vi "ZeroMQ_FOC_REQREP.vi"() -> ()   [LabVIEW 2018]
uses:
  <vilib>/addons/zeromq/socket_type.ctl
  <vilib>/addons/zeromq/socket_options.ctl
  <vilib>/addons/zeromq/zeromq.lvlib
  <vilib>/addons/zeromq/zmq_socket.lvclass
  <vilib>/addons/zeromq/zmq_context.lvclass
panel:
  out "error out 3":errorcluster
  out "error out 4":errorcluster
  in  "stop 4":bool
  out "command 2":string
  out "reply":string
  out "error out 2":errorcluster
  out "message":string
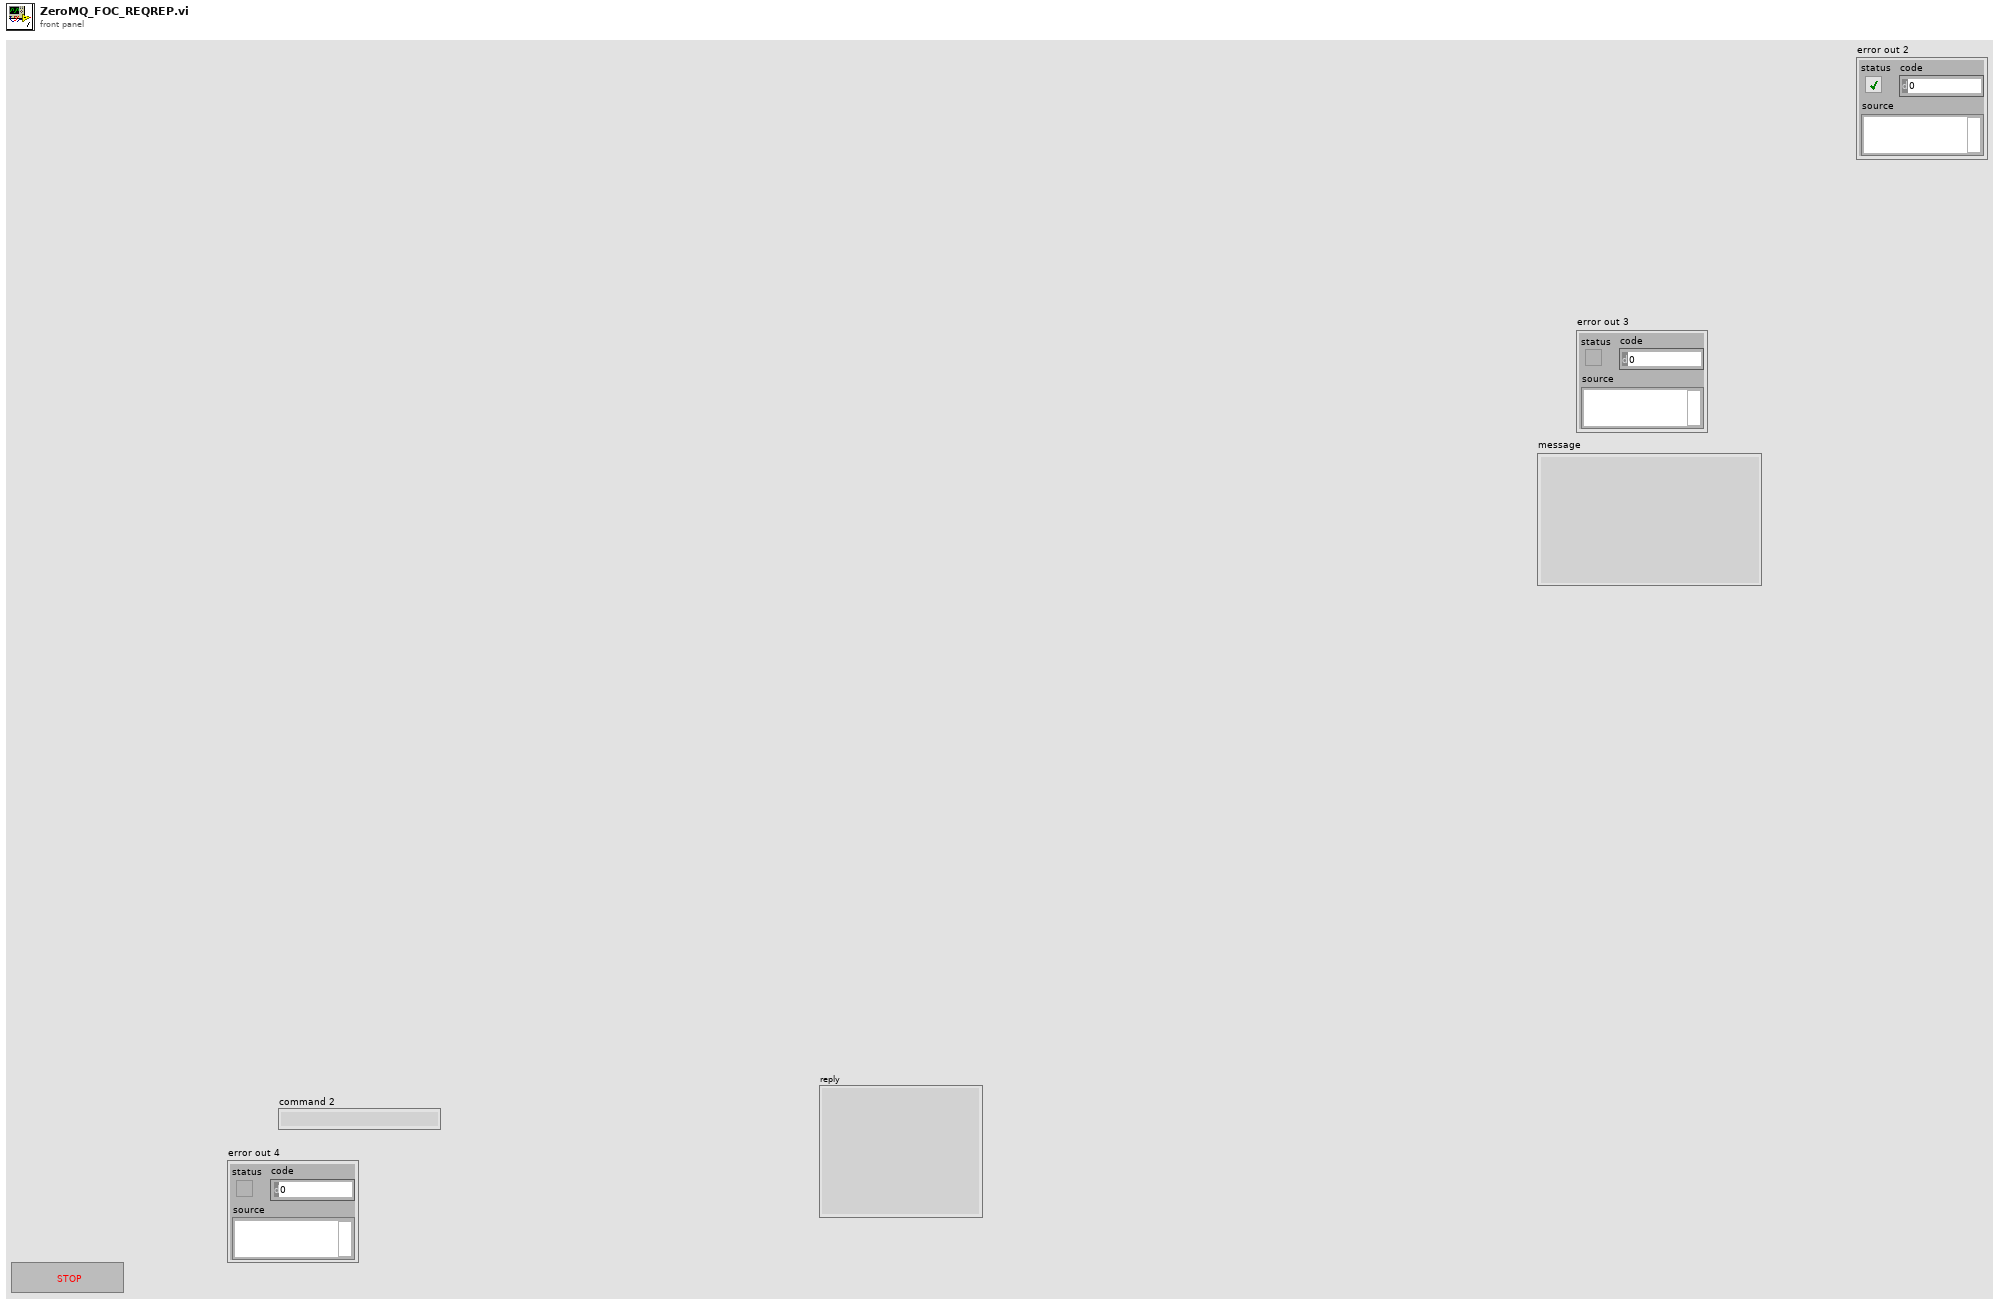
[diagram p1: front panel]
types:
  T1 = typedef "zeromq.lvlib/socket_options.ctl" = enum8{"NONE", "ZMQ_HWM", "<2>", "ZMQ_SWAP", "ZMQ_AFFINITY", "ZMQ_ROUTING_ID", "ZMQ_SUBSCRIBE", "ZMQ_UNSUBSCRIBE", "ZMQ_RATE", "ZMQ_RECOVERY_IVL", "ZMQ_MCAST_LOOP", "ZMQ_SNDBUF", "ZMQ_RCVBUF", "ZMQ_RCVMORE", "ZMQ_FD", "ZMQ_EVENTS", "ZMQ_TYPE", "ZMQ_LINGER", "ZMQ_RECONNECT_IVL", "ZMQ_BACKLOG", "ZMQ_RECOVERY_IVL_MSEC", "ZMQ_RECONNECT_IVL_MAX", "ZMQ_MAXMSGSIZE", "ZMQ_SNDHWM", "ZMQ_RCVHWM", "ZMQ_MULTICAST_HOPS", "<26>", "ZMQ_RCVTIMEO", "ZMQ_SNDTIMEO", "<29>", "<30>", "ZMQ_IPV4ONLY", "ZMQ_LAST_ENDPOINT", "ZMQ_ROUTER_MANDATORY", "ZMQ_TCP_KEEPALIVE", "ZMQ_TCP_KEEPALIVE_CNT", "ZMQ_TCP_KEEPALIVE_IDLE", "ZMQ_TCP_KEEPALIVE_INTVL", "ZMQ_TCP_ACCEPT_FILTER", "ZMQ_IMMEDIATE", "ZMQ_XPUB_VERBOSE", "ZMQ_ROUTER_RAW", "ZMQ_IPV6", "ZMQ_MECHANISM", "ZMQ_PLAIN_SERVER", "ZMQ_PLAIN_USERNAME", "ZMQ_PLAIN_PASSWORD", "ZMQ_CURVE_SERVER", "ZMQ_CURVE_PUBLICKEY", "ZMQ_CURVE_SECRETKEY", "ZMQ_CURVE_SERVERKEY", "ZMQ_PROBE_ROUTER", "ZMQ_REQ_CORRELATE", "ZMQ_REQ_RELAXED", "ZMQ_CONFLATE", "ZMQ_ZAP_DOMAIN", "ZMQ_ROUTER_HANDOVER", "ZMQ_TOS", "ZMQ_IPC_FILTER_PID", "ZMQ_IPC_FILTER_UID", "ZMQ_IPC_FILTER_GID", "ZMQ_CONNECT_ROUTING_ID", "ZMQ_GSSAPI_SERVER", "ZMQ_GSSAPI_PRINCIPAL", "ZMQ_GSSAPI_SERVICE_PRINCIPAL", "ZMQ_GSSAPI_PLAINTEXT", "ZMQ_HANDSHAKE_IVL", "<67>", "ZMQ_SOCKS_PROXY", "ZMQ_XPUB_NODROP", "ZMQ_BLOCKY", "ZMQ_XPUB_MANUAL", "ZMQ_XPUB_WELCOME_MSG", "ZMQ_STREAM_NOTIFY", "ZMQ_INVERT_MATCHING", "ZMQ_HEARTBEAT_IVL", "ZMQ_HEARTBEAT_TTL", "ZMQ_HEARTBEAT_TIMEOUT", "ZMQ_XPUB_VERBOSER", "ZMQ_CONNECT_TIMEOUT", "ZMQ_TCP_MAXRT", "ZMQ_THREAD_SAFE", "<82>", "<83>", "ZMQ_MULTICAST_MAXTPDU", "ZMQ_VMCI_BUFFER_SIZE", "ZMQ_VMCI_BUFFER_MIN_SIZE", "ZMQ_VMCI_BUFFER_MAX_SIZE", "ZMQ_VMCI_CONNECT_TIMEOUT", "ZMQ_USE_FD", "ZMQ_GSSAPI_PRINCIPAL_NAMETYPE", "ZMQ_GSSAPI_SERVICE_PRINCIPAL_NAMETYPE", "ZMQ_BINDTODEVICE", "ZMQ_ZAP_ENFORCE_DOMAIN", "ZMQ_LOOPBACK_FASTPATH", "ZMQ_METADATA", "ZMQ_MULTICAST_LOOP", "ZMQ_ROUTER_NOTIFY"}
  T2 = typedef "zeromq.lvlib/socket_type.ctl" = enum8{"ZMQ_PAIR", "ZMQ_PUB", "ZMQ_SUB", "ZMQ_REQ", "ZMQ_REP", "ZMQ_DEALER", "ZMQ_ROUTER", "ZMQ_PULL", "ZMQ_PUSH", "ZMQ_XPUB", "ZMQ_XSUB", "ZMQ_STREAM", "ZMQ_SERVER", "ZMQ_CLIENT", "ZMQ_RADIO", "ZMQ_DISH", "ZMQ_GATHER", "ZMQ_SCATTER", "ZMQ_DGRAM"}
  T3 = cluster{"ID":u32, "Address":string, "Service Name 1":string, "Service Name 2":string, "queue TX":refnum<queue>, "queue RX":refnum<queue>, "Port 1":u32, "Port 2":u32}
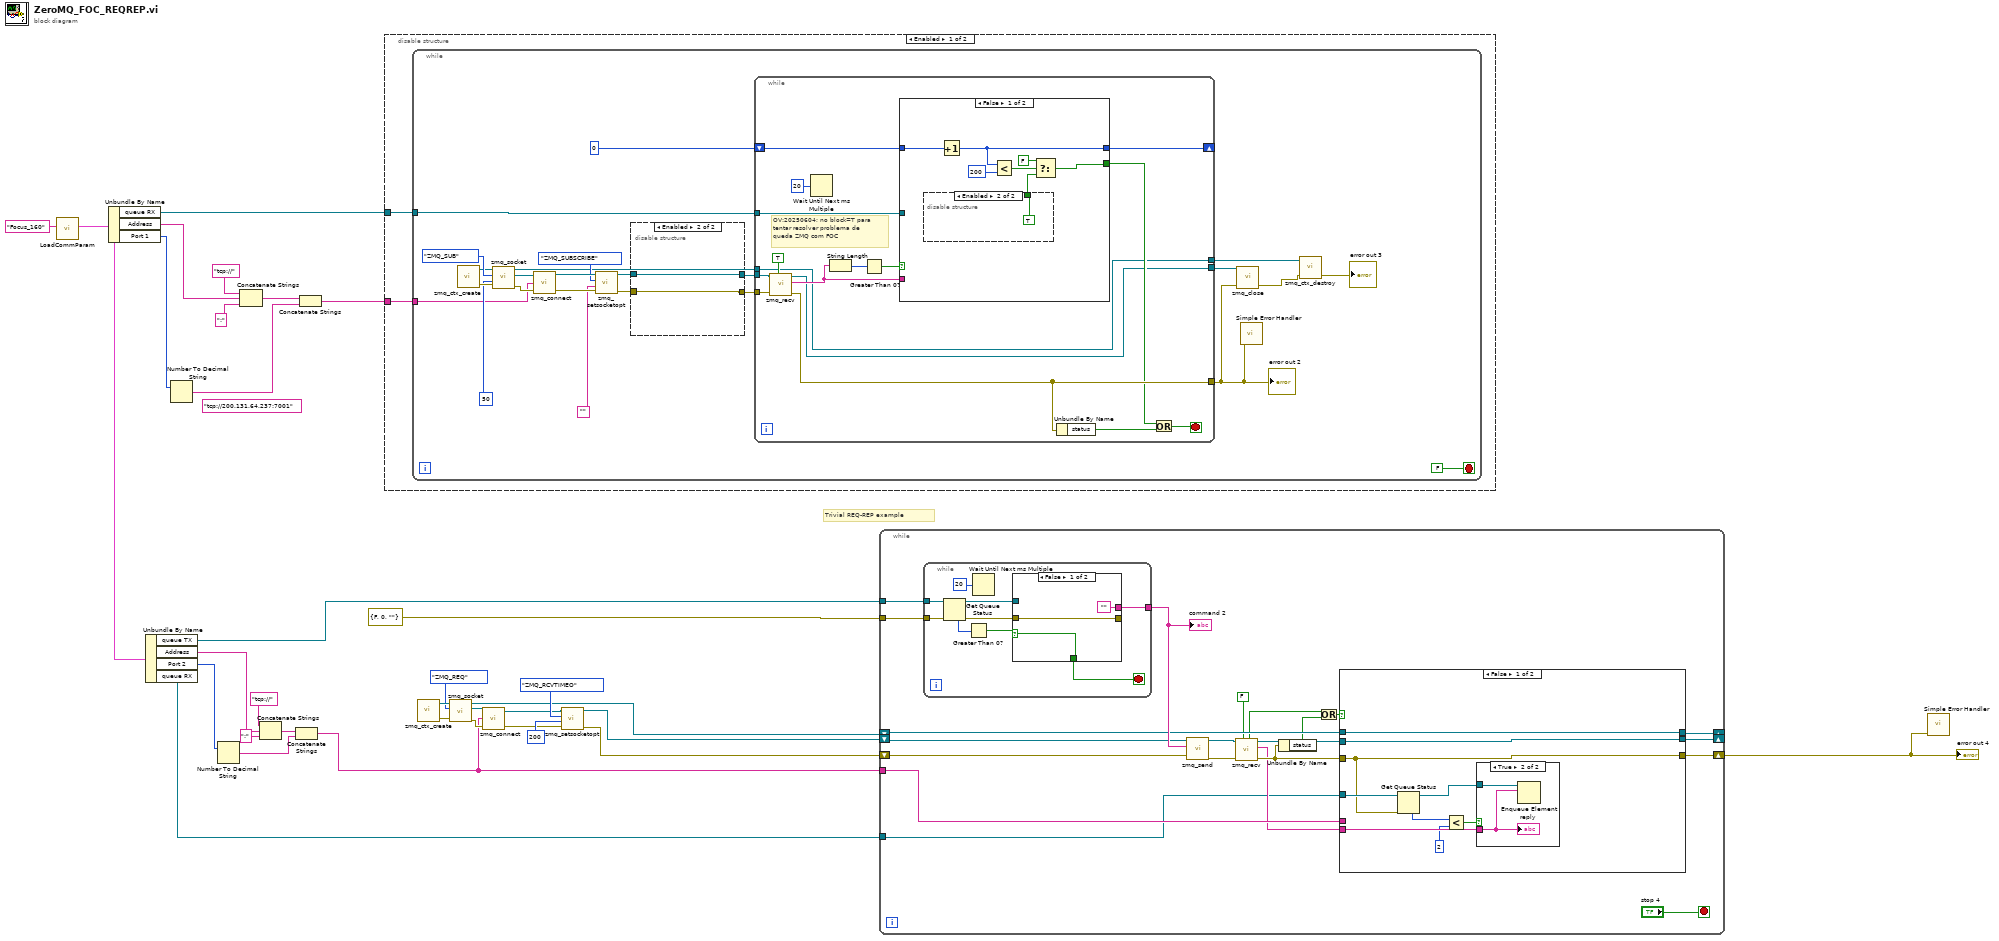
[diagram p0: block diagram]
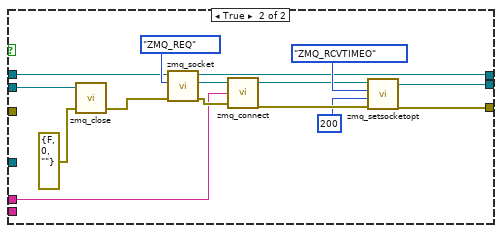
[diagram p3: hidden frame]
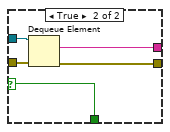
[diagram p4: hidden frame]
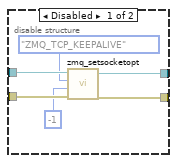
[diagram p5: hidden frame]
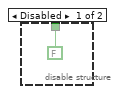
[diagram p6: hidden frame]
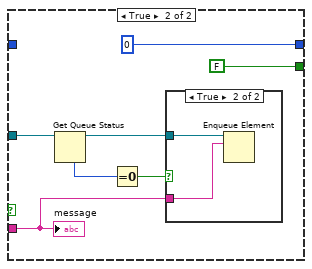
[diagram p7: hidden frame]
diagram:
  (unwired) "tcp://200.131.64.237:7001" ("endpoint")
  # "Trivial REQ-REP example"
  n1 = call "LoadCommParam.vi"("section name"="Focus_160") -> ("output cluster"=w1:T3)  [unwired: 10 in]
  n2 = Unbundle By Name(w1) -> ("queue RX"=w25:refnum<queue>, "Address"=w32:string, "Port 1"=w31:u32)
  n3 = Unbundle By Name(w1) -> ("queue TX"=w16:refnum<queue>, "Address"=w18:string, "Port 2"=w17:u32, "queue RX"=w2:refnum<queue>)
  n4 = Number To Decimal String(number=w31) -> (decimal integer string=w30:string)  [unwired: 1 in]
  n5 = Number To Decimal String(number=w17) -> (decimal integer string=w22:string)  [unwired: 1 in]
  n6 = Concatenate Strings("tcp://" ("string"), w32, ":" ("string")) -> (w29:string)
  n7 = Concatenate Strings("tcp://" ("string"), w18, ":" ("string")) -> (w21:string)
  n8 = Concatenate Strings(w21, w22) -> (w10:string)
  n9 = Concatenate Strings(w29, w30) -> (w26:string)
  n10 = disable-structure shown="Enabled" {
    disable-tunnel: w25 -> [w35 _]
    disable-tunnel: w26 -> [w34 _]
    frame Enabled {
      n11 = while {
        tunnel: w35 -> [w50]
        tunnel: w34 -> [w49]
        stop <- FALSE stop-if-true
        n12 = call <vilib>:"zmq_ctx_create.vi"() -> ("error out"=w58:errorcluster, "context out"=w52:refnum<class "zmq_context.lvclass">)  [unwired: 4 in]
        n13 = call <vilib>:"zmq_socket.vi"("error in"=w58, "linger (ms)"=50, "socket type"=socket_type."ZMQ_SUB", "context in"=w52) -> ("error out"=w57:errorcluster, "socket out"=w53:refnum<class "zmq_socket.lvclass">, "context out"=w41:refnum<class "zmq_context.lvclass">)  [unwired: 1 in]
        n14 = call <vilib>:"zmq_connect.vi"("error in"=w57, "endpoint"=w49, "socket in"=w53) -> ("error out"=w55:errorcluster, "socket out"=w56:refnum<class "zmq_socket.lvclass">)  [unwired: 1 in]
        n15 = call <vilib>:"zmq_setsocketopt.vi"("error in"=w55, "value"="", "option"=socket_options."ZMQ_SUBSCRIBE", "socket in"=w56) -> ("error out"=w44:errorcluster, "socket out"=w46:refnum<class "zmq_socket.lvclass">)  [unwired: 2 in]
        n16 = disable-structure shown="Enabled" {
          disable-tunnel: w46 -> [w65 w67]
          disable-tunnel: [w64 w67] -> w45
          disable-tunnel: w44 -> [w63 w66]
          disable-tunnel: [w62 w66] -> w43
          frame Disabled {
            n17 = call <vilib>:"zmq_setsocketopt.vi"("error in"=w63, "value"=-1, "option"=socket_options."ZMQ_TCP_KEEPALIVE", "socket in"=w65) -> ("error out"=w62:errorcluster, "socket out"=w64:refnum<class "zmq_socket.lvclass">)  [unwired: 2 in]
          }
          frame Enabled {
          }
        }
        n18 = while {
          tunnel: w45 -> [w82]
          tunnel: w43 -> [w83]
          tunnel: [w73] -> w38
          tunnel: w50 -> [w79]
          shift-right: [w74] -> _
          shift-left: 0 -> [w75]
          tunnel: [w69] -> w40
          tunnel: w41 -> [w68]
          tunnel: [w68] -> w39
          stop <- w70 stop-if-true
          # "OV:20250604; no block=T para\ntentar resolver problema de\nqueda ZMQ com FOC"
          n19 = call <vilib>:"zmq_recv.vi"("no block? (F)"=TRUE, "error in"=w83, "socket in"=w82) -> ("error out"=w73:errorcluster, "data"=w78:string, "socket out"=w69:refnum<class "zmq_socket.lvclass">)  [unwired: 2 in, 2 out]
          n20 = Wait Until Next ms Multiple(millisecond multiple=u32 20) -> ()  [unwired: 1 out]
          n21 = String Length(string=w78) -> (length=w81:i32)
          n22 = Greater Than 0?(x=w81) -> (x > 0?=w80:bool)
          n23 = case shown="False" w80 {
            tunnel: w79 -> [_ w98]
            tunnel: w78 -> [_ w95]
            tunnel: w75 -> [w90 _]
            tunnel: [w89 0] -> w74
            tunnel: [w86 FALSE] -> w71
            frame False {
              n24 = disable-structure shown="Enabled" {
                disable-tunnel: [FALSE ("f") TRUE] -> w84
                frame Disabled {
                }
                frame Enabled {
                }
              }
              n25 = Increment(x=w90) -> (x+1=w89:i32)
              n26 = Less?(x=w89, y=200) -> (x < y?=w87:bool)
              n27 = Select(t=FALSE, s=w87, f=w84) -> (s? t:f=w86:bool)
            }
            frame True {
              n28 = Get Queue Status(queue=w98) -> (queue out=w96:refnum<queue>, # elements in queue=w99:i32)  [unwired: 2 in, 6 out]
              n29 = Equal To 0?(x=w99) -> (x = 0?=w97:bool)
              n30 = case shown="True" w97 {
                tunnel: w96 -> [_ w101]
                tunnel: w95 -> [_ w100]
                frame False {
                }
                frame True {
                  n31 = Enqueue Element(queue=w101, element=w100) -> ()  [unwired: 2 in, 3 out]
                }
              }
              "message" <- w95
            }
          }
          n32 = Unbundle By Name(w73) -> ("status"=w72:bool)
          n33 = Or(x=w71, y=w72) -> (x .or. y?=w70:bool)
        }
        "error out 2" <- w38
        n34 = call <vilib>:"zmq_close.vi"("error in"=w38, "socket"=w40) -> ("error out"=w37:errorcluster)  [unwired: 3 in]
        n35 = call <vilib>:"Simple Error Handler.vi"("error in (no error)"=w38) -> ()  [unwired: 4 in, 5 out]
        n36 = call <vilib>:"zmq_ctx_destroy.vi"("error in"=w37, "context in"=w39) -> ("error out"=→"error out 3":errorcluster)  [unwired: 3 in]
      }
    }
    frame Disabled {
    }
  }
  n37 = call <vilib>:"zmq_ctx_create.vi"() -> ("error out"=w15:errorcluster, "context out"=w12:refnum<class "zmq_context.lvclass">)  [unwired: 4 in]
  n38 = call <vilib>:"zmq_socket.vi"("error in"=w15, "socket type"=socket_type."ZMQ_REQ", "context in"=w12) -> ("error out"=w13:errorcluster, "socket out"=w14:refnum<class "zmq_socket.lvclass">, "context out"=w5:refnum<class "zmq_context.lvclass">)  [unwired: 2 in]
  n39 = call <vilib>:"zmq_connect.vi"("error in"=w13, "endpoint"=w10, "socket in"=w14) -> ("error out"=w6:errorcluster, "socket out"=w7:refnum<class "zmq_socket.lvclass">)  [unwired: 1 in]
  n40 = call <vilib>:"zmq_setsocketopt.vi"("error in"=w6, "value"=200 ("max queue size (-1, unlimited)"), "option"=socket_options."ZMQ_RCVTIMEO", "socket in"=w7) -> ("error out"=w3:errorcluster, "socket out"=w4:refnum<class "zmq_socket.lvclass">)  [unwired: 2 in]
  n41 = while {
    tunnel: w16 -> [w122]
    tunnel: errorcluster {"status"=FALSE, "code"=0, "source"=""} ("error out") -> [w118]
    tunnel: w10 -> [w107]
    shift-right: [w106] -> _
    shift-left: w5 -> [w117]
    shift-right: [w105] -> _
    shift-left: w4 -> [w116]
    shift-right: [w119] -> w24
    shift-left: w3 -> [w104]
    tunnel: w2 -> [w102]
    stop <- "stop 4" stop-if-true
    n42 = while {
      tunnel: w122 -> [w156]
      tunnel: w118 -> [w155]
      tunnel: [w151] -> w121
      stop <- w150 stop-if-true
      n43 = Get Queue Status(queue=w156, error in (no error)=w155) -> (queue out=w152:refnum<queue>, error out=w153:errorcluster, # elements in queue=w157:i32)  [unwired: 1 in, 5 out]
      n44 = Greater Than 0?(x=w157) -> (x > 0?=w154:bool)
      n45 = Wait Until Next ms Multiple(millisecond multiple=u32 20) -> ()  [unwired: 1 out]
      n46 = case shown="False" w154 {
        selector: w154 -> [w158 w161]
        tunnel: w153 -> [w160 w165]
        tunnel: w152 -> [_ w164]
        tunnel: [w160 w163] -> _
        tunnel: ["" w162] -> w151
        tunnel: [w158 w161] -> w150
        frame False {
        }
        frame True {
          n47 = Dequeue Element(queue=w164, error in (no error)=w165) -> (element=w162:string, error out=w163:errorcluster)  [unwired: 1 in, 2 out]
        }
      }
    }
    "command 2" <- w121
    n48 = call <vilib>:"zmq_send.vi"("error in"=w104, "data"=w121, "socket in"=w116) -> ("error out"=w114:errorcluster, "socket out"=w115:refnum<class "zmq_socket.lvclass">)  [unwired: 4 in]
    n49 = call <vilib>:"zmq_recv.vi"("no block? (F)"=FALSE, "error in"=w114, "socket in"=w115) -> ("error out"=w109:errorcluster, "data"=w103:string, "socket out"=w108:refnum<class "zmq_socket.lvclass">, "timeout?"=w110:bool)  [unwired: 2 in, 1 out]
    n50 = Unbundle By Name(w109) -> ("status"=w111:bool)
    n51 = Or(x=w110, y=w111) -> (x .or. y?=w112:bool)
    n52 = case shown="False" w112 {
      tunnel: [w126 w136] -> w119
      tunnel: w117 -> [w130 w138]
      tunnel: w109 -> [w126 _]
      tunnel: w108 -> [w131 w139]
      tunnel: w107 -> [_ w137]
      tunnel: [w131 w135] -> w105
      tunnel: [w130 w134] -> w106
      tunnel: w103 -> [w128 _]
      tunnel: w102 -> [w127 _]
      frame False {
        n53 = Get Queue Status(queue=w127, error in (no error)=w126) -> (queue out=w129:refnum<queue>, # elements in queue=w124:i32)  [unwired: 1 in, 6 out]
        n54 = Less?(x=w124, y=2) -> (x < y?=w125:bool)
        n55 = case shown="True" w125 {
          tunnel: w129 -> [_ w133]
          tunnel: w128 -> [_ w132]
          frame False {
          }
          frame True {
            n56 = Enqueue Element(queue=w133, element=w132) -> ()  [unwired: 2 in, 3 out]
            "reply" <- w132
          }
        }
      }
      frame True {
        n57 = call <vilib>:"zmq_close.vi"("error in"=errorcluster {"status"=FALSE, "code"=0, "source"=""}, "socket"=w139) -> ("error out"=w141:errorcluster)  [unwired: 3 in]
        n58 = call <vilib>:"zmq_socket.vi"("error in"=w141, "socket type"=socket_type."ZMQ_REQ", "context in"=w138) -> ("error out"=w147:errorcluster, "socket out"=w148:refnum<class "zmq_socket.lvclass">, "context out"=w134:refnum<class "zmq_context.lvclass">)  [unwired: 2 in]
        n59 = call <vilib>:"zmq_connect.vi"("error in"=w147, "endpoint"=w137, "socket in"=w148) -> ("error out"=w143:errorcluster, "socket out"=w144:refnum<class "zmq_socket.lvclass">)  [unwired: 1 in]
        n60 = call <vilib>:"zmq_setsocketopt.vi"("error in"=w143, "value"=200 ("max queue size (-1, unlimited)"), "option"=socket_options."ZMQ_RCVTIMEO", "socket in"=w144) -> ("error out"=w136:errorcluster, "socket out"=w135:refnum<class "zmq_socket.lvclass">)  [unwired: 2 in]
      }
    }
  }
  "error out 4" <- w24
  n61 = call <vilib>:"Simple Error Handler.vi"("error in (no error)"=w24) -> ()  [unwired: 4 in, 5 out]
